vi "Chain6.vi"(7 "Name (\"\" to Use UUID)":string="CSM-Module") -> ()   [LabVIEW 2017, in "CSM-Testcase.lvlib"]
doc: "Creates a template for a CSM module without a user interface.\n\n> [!NOTE] CSM Name Rules\n> - The CSM module name must be unique to avoid entering the \"Critical Error\" state.\n> - If the input is \"\", a UUID will be used as the module name. This module will operate in independent mode and will not be listed in the module list.\n> - If the input ends with '#', the module will run in work mode. Modules with the same name will share the same message queue. External messages will be handled by the idle module.\n\n> [!NOTE] CSM Initialization State\n> - The default value is \"Macro: Initialize\", consistent with the JKISM state machine.\n> - This state is typically not modified and is provided to facilitate external programmatic changes to the initialization state.\n\n\n-- <b>Controls</b> --\n- <b>Name (\"\" to Use UUID)</b>: CSM Module Name\n- <b>Init State(\"Macro: Initialize\")</b>: Initialization State, default is \"Macro: Initialize\""
uses:
  CSM-Testcase.lvlib
  src/user.lib/_NEVSTOP/Communicable State Machine(CSM)/AdvanceAPI/CSM - Revert Arguments-Safe String.vi
  src/user.lib/_NEVSTOP/Communicable State Machine(CSM)/AdvanceAPI/CSM - Make String Arguments Safe.vi
  src/user.lib/_NEVSTOP/Communicable State Machine(CSM)/AdvanceAPI/CSM - Break Down Multiple States String.vi
  src/user.lib/_NEVSTOP/Communicable State Machine(CSM)/AdvanceAPI/CSM - Keywords.vi
  src/user.lib/_NEVSTOP/Communicable State Machine(CSM)/_Shared/Trim Single-line Text.vi
  src/user.lib/_NEVSTOP/Communicable State Machine(CSM)/_Polymophic/Build No-Reply Asynchronous Message with Arguments.vi
  src/user.lib/_NEVSTOP/Communicable State Machine(CSM)/_Polymophic/Build Asynchronous Message with Arguments.vi
  src/user.lib/_NEVSTOP/Communicable State Machine(CSM)/_Polymophic/Build Register Message.vi
  src/user.lib/_NEVSTOP/Communicable State Machine(CSM)/_Polymophic/Build Interrupt Broadcast Message.vi
  src/user.lib/_NEVSTOP/Communicable State Machine(CSM)/Communicable State Machine.lvlib
panel:
  out "Error Occurred":errorcluster
  out "State History":string
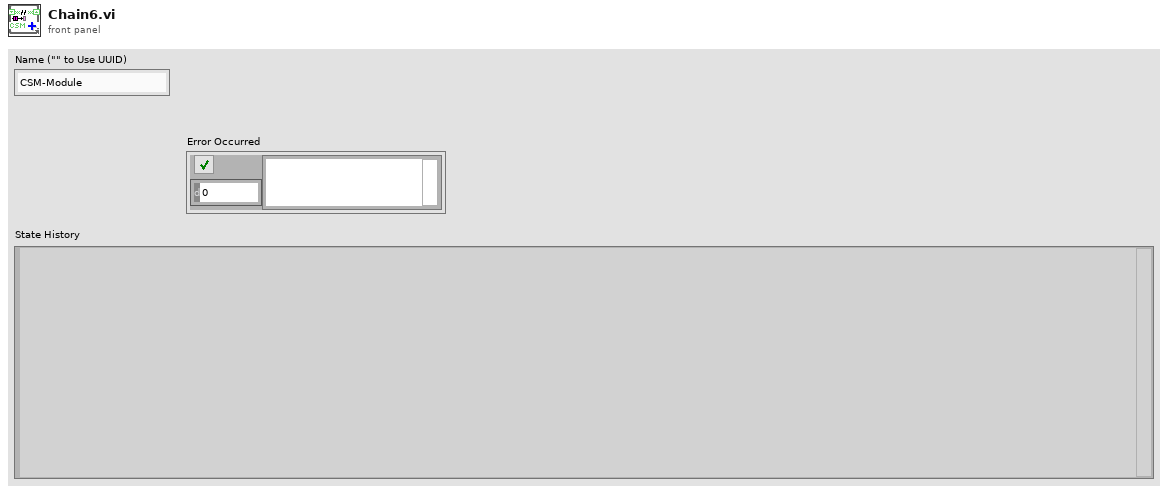
[diagram p1: front panel]
types:
  T1 = cluster{"Arguments":string, "Response":string, "error":errorcluster}
  T2 = enum32{"Invalid", "Standard", "Closed", "Hidden", "Minimized", "Maximized"}
  T3 = enum32{"invalid app kind", "Development System", "Run Time System", "Student Edition", "Embedded LabVIEW", "Evaluation", "Custom"}
  T4 = typedef "Communicable State Machine.lvlib/_CSM_Response Source Message.ctl" = cluster{"‘State":string, "’Arguments":string, "’Error":errorcluster}
  T5 = cluster{"Current VI Reference":refnum<vi>, "Close Panel on Exit?":bool}
  T6 = cluster{"Core":cluster{"Current VI Reference":refnum<vi>, "Close Panel on Exit?":bool}, "Your Boolean data":bool, "Your string data":string, "Counter":u32}
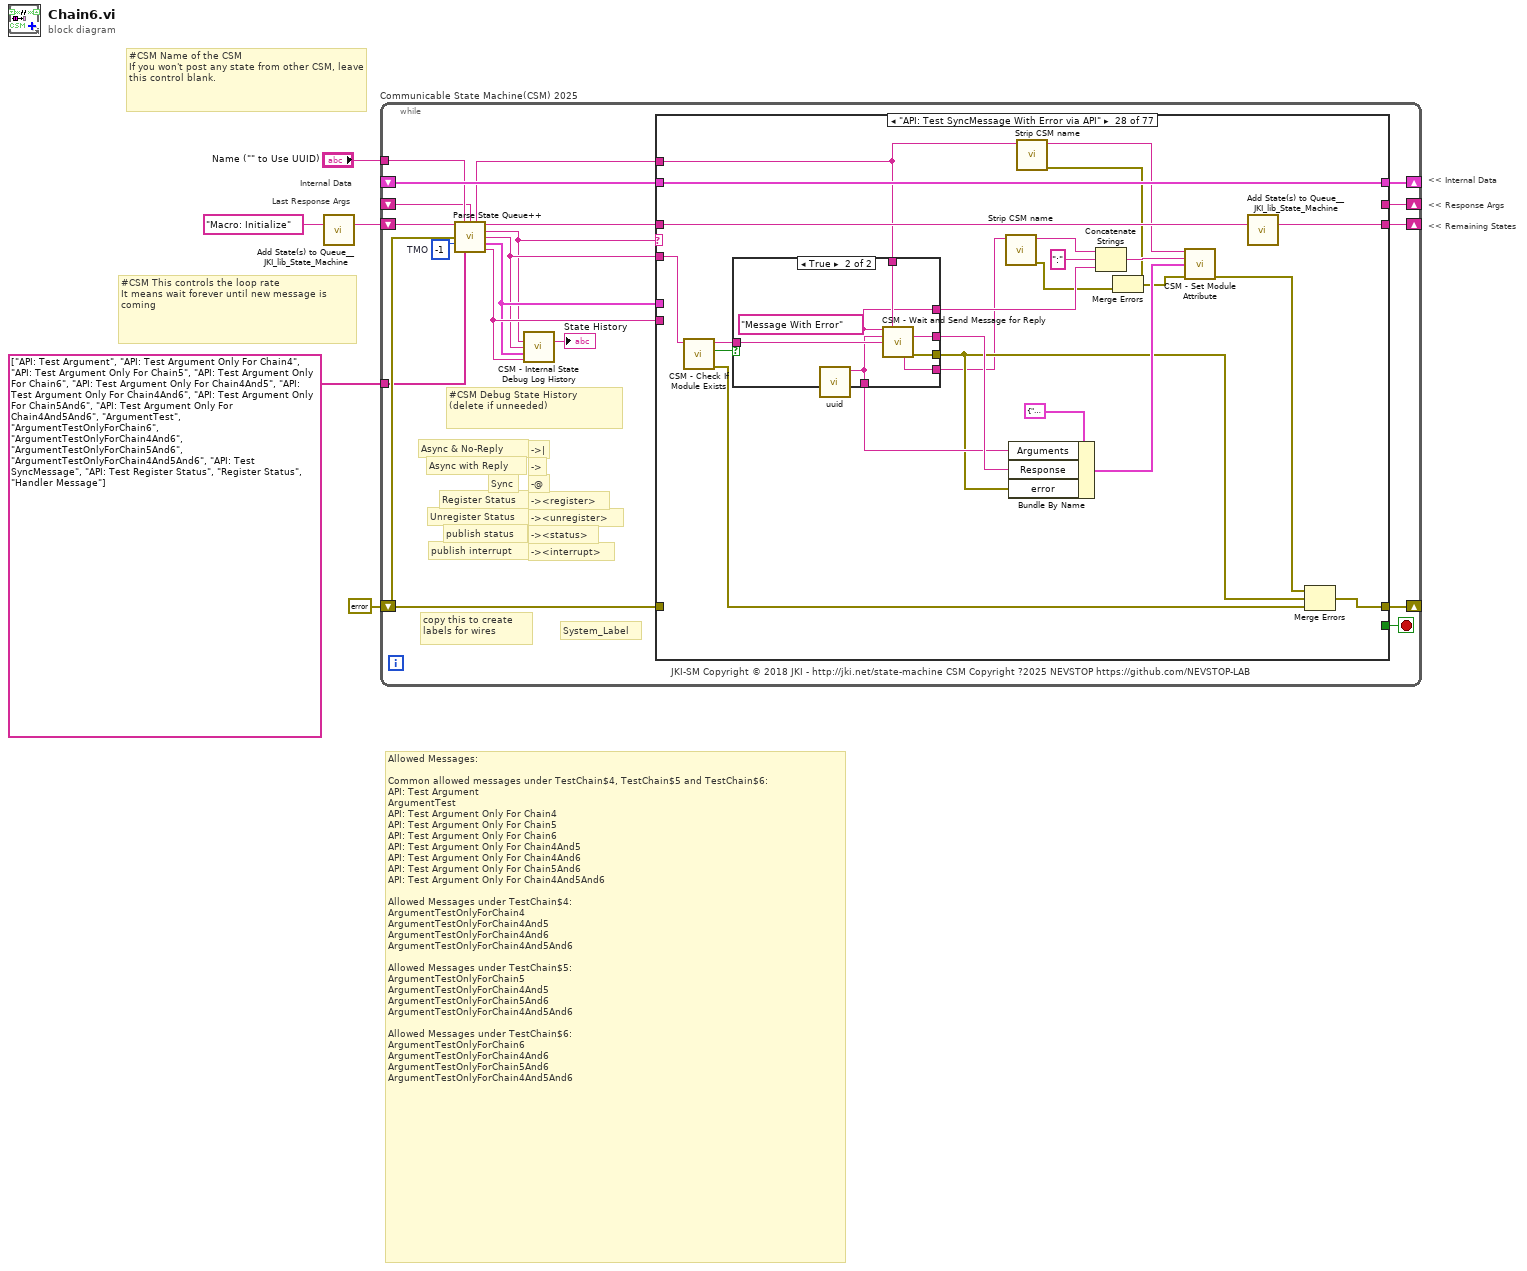
[diagram p0: block diagram]
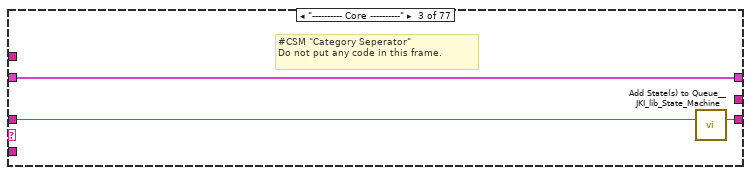
[diagram p4: hidden frame]
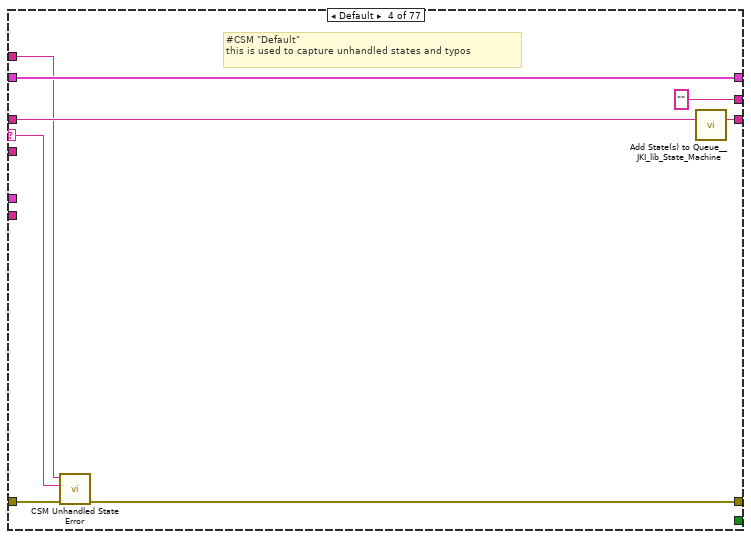
[diagram p5: hidden frame]
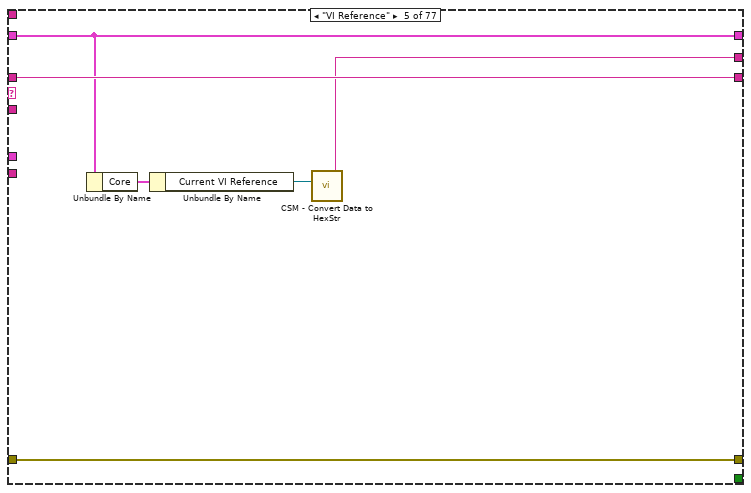
[diagram p6: hidden frame]
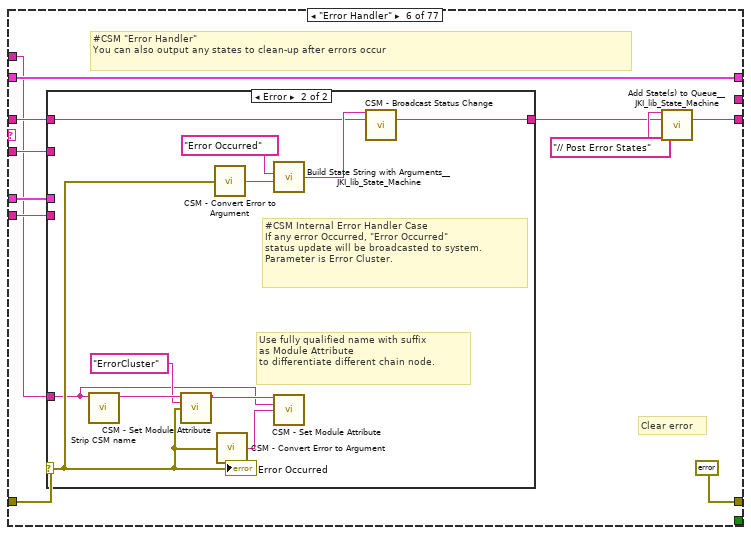
[diagram p7: hidden frame]
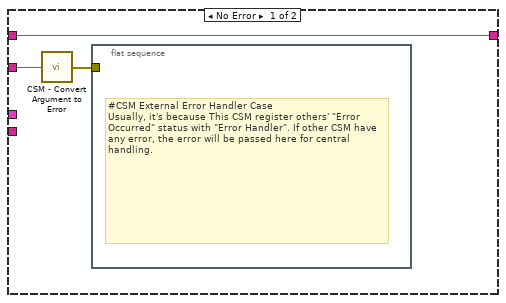
[diagram p8: hidden frame]
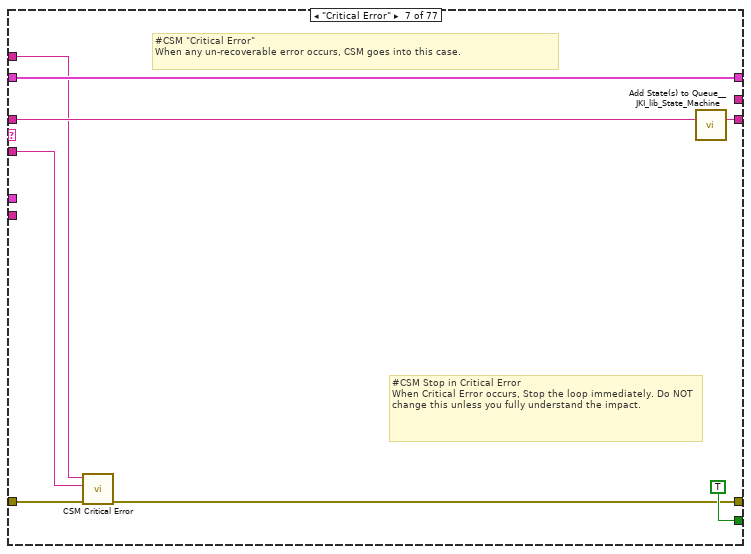
[diagram p9: hidden frame]
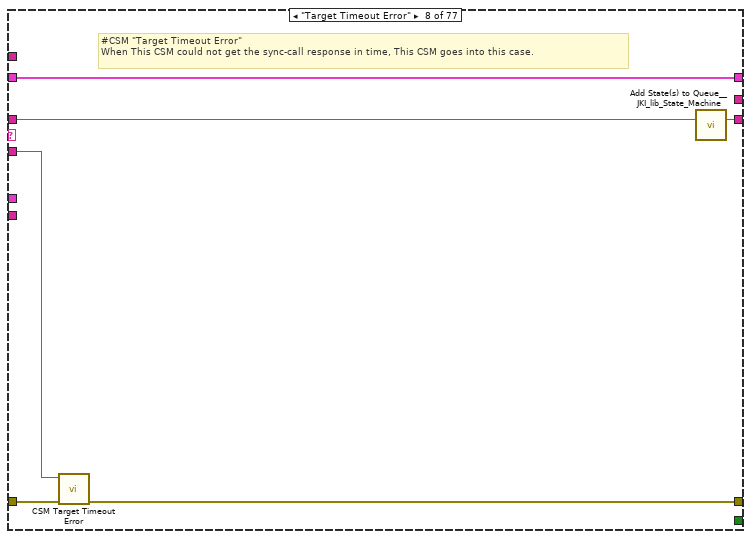
[diagram p10: hidden frame]
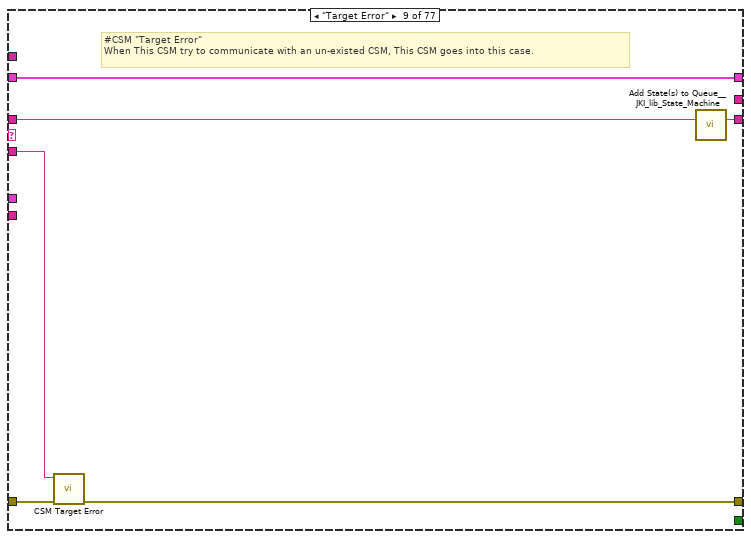
[diagram p11: hidden frame]
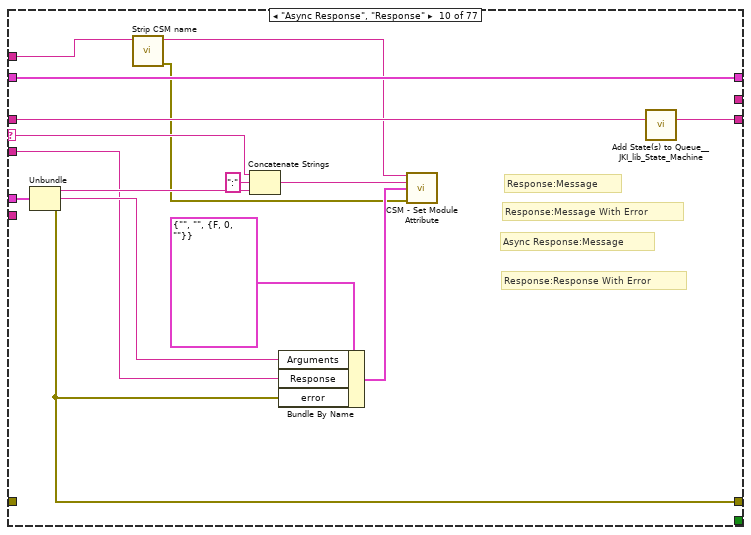
[diagram p12: hidden frame]
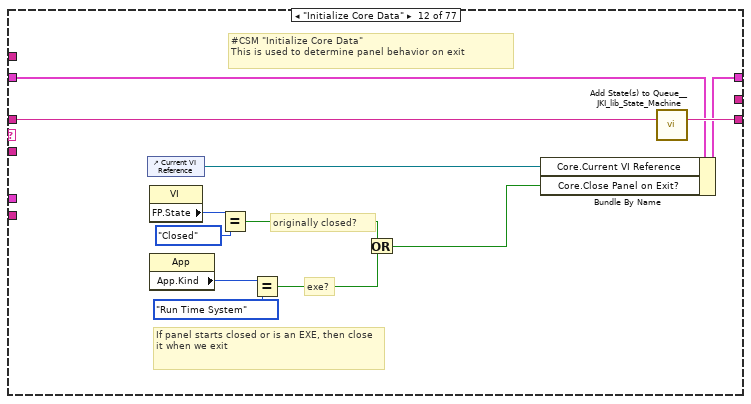
[diagram p14: hidden frame]
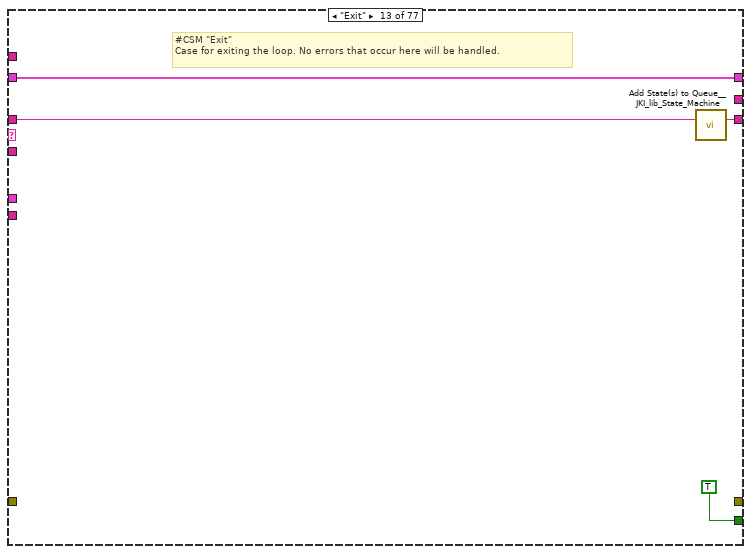
[diagram p15: hidden frame]
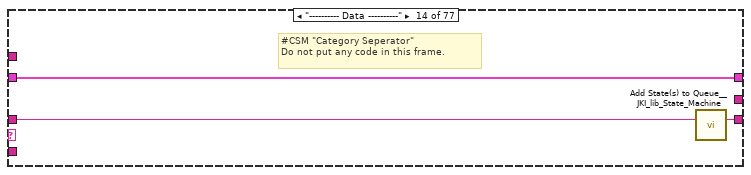
[diagram p16: hidden frame]
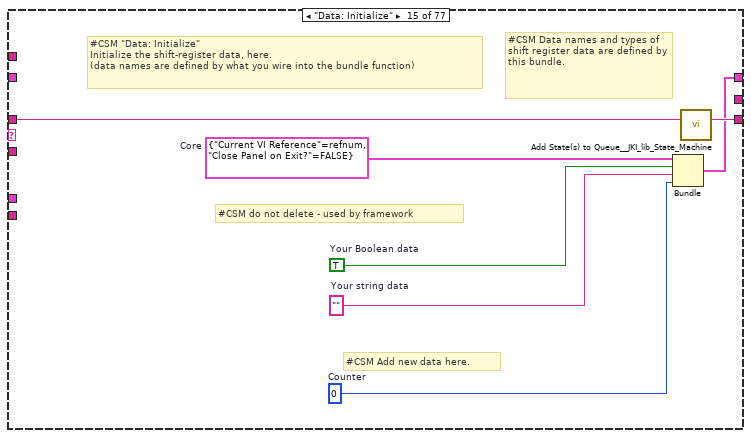
[diagram p17: hidden frame]
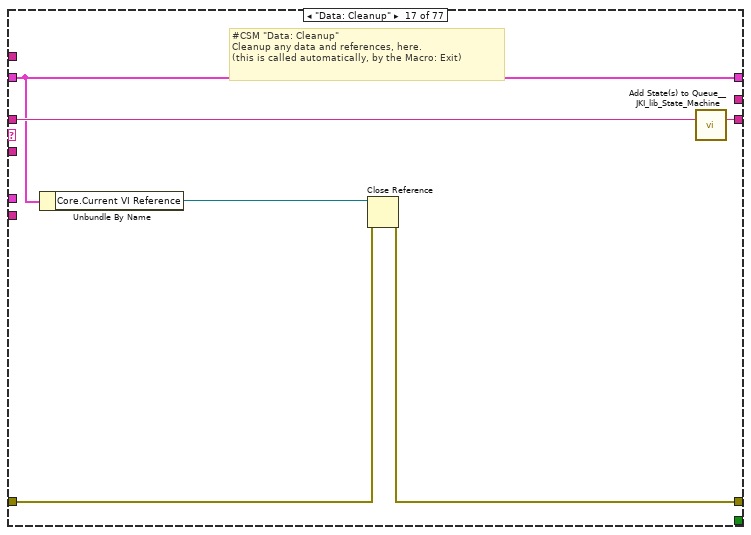
[diagram p19: hidden frame]
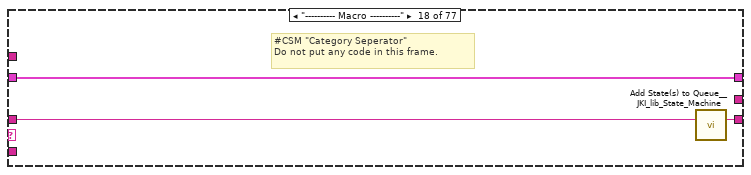
[diagram p20: hidden frame]
diagram:
  # "Allowed Messages:\n\nCommon allowed messages under TestChain$4, TestChain$5 and TestChain$6:\nAPI: Test Argument\nArgumentTest\nAPI: Test Argument Only For Chain4\nAPI: Test Argument Only For Chain5\nAPI: Test Argument Only For Chain6\nAPI: Test Argument Only For Chain4And5\nAPI: Test Argument Only For Chain4And6\nAPI: Test Argument Only For Chain5And6\nAPI: Test Argument Only For Chain4And5And6\n\nAllowed Messages under TestChain$4:\nArgumentTestOnlyForChain4\nArgumentTestOnlyForChain4And5\nArgumentTestOnlyForChain4And6\nArgumentTestOnlyForChain4And5And6\n\nAllowed Messages under TestChain$5:\nArgumentTestOnlyForChain5\nArgumentTestOnlyForChain4And5\nArgumentTestOnlyForChain5And6\nArgumentTestOnlyForChain4And5And6\n\nAllowed Messages under TestChain$6:\nArgumentTestOnlyForChain6\nArgumentTestOnlyForChain4And6\nArgumentTestOnlyForChain5And6\nArgumentTestOnlyForChain4And5And6"
  # "Last Response Args"
  # "Internal Data"
  # "#CSM Name of the CSM\nIf you won't post any state from other CSM, leave this control blank."
  # "#CSM This controls the loop rate\nIt means wait forever until new message is coming"
  # "<< Internal Data"
  # "<< Response Args"
  # "<< Remaining States"
  n1 = call <vilib>:"Add State(s) to Queue__JKI_lib_State_Machine.vi"("State(s) in (\"\")"="Macro: Initialize" ("Init State(\"Macro: Initialize\")")) -> ("States Out"=w5:string)  [unwired: 14 in]
  n2 = while "Communicable State Machine(CSM) 2025" {
    shift-right: [w19] -> _
    shift-left: _ -> [w18]
    shift-right: [w22] -> _
    shift-left: errorcluster {"status"=FALSE, "code"=0, "source"=""} ("error out") -> [w8]
    shift-right: [w21] -> _
    shift-left: w5 -> [w23]
    tunnel: "Name (\"\" to Use UUID)" -> [w15]
    shift-right: [w16] -> _
    shift-left: _ -> [w10]
    tunnel: string[] ["API: Test Argument", "API: Test Argument Only For Chain4", "API: Test Argument Only For Chain5", "API: Test Argument Only For Chain6", "API: Test Argument Only For Chain4And5", "API: Test Argument Only For Chain4And6", "API: Test Argument Only For Chain5And6", "API: Test Argument Only For Chain4And5And6", "ArgumentTest", "ArgumentTestOnlyForChain6", "ArgumentTestOnlyForChain4And6", "ArgumentTestOnlyForChain5And6", "ArgumentTestOnlyForChain4And5And6", "API: Test SyncMessage", "API: Test Register Status", "Register Status", "Handler Message"] ("Allowed Messages (Empty for All)") -> [w6]
    stop <- w20 stop-if-true
    w17 = -1  # TMO
    # "#CSM Debug State History\n(delete if unneeded)"
    # "-><interrupt>"
    # "-><status>"
    # "-><unregister>"
    # "-><register>"
    # "-@"
    # "->"
    # "->|"
    # "publish interrupt"
    # "publish status"
    # "Unregister Status"
    # "Register Status"
    # "Sync"
    # "Async with Reply"
    # "Async & No-Reply"
    # "JKI-SM Copyright © 2018 JKI - http://jki.net/state-machine CSM Copyright ?2025 NEVSTOP https://github.com/NEVSTOP-LAB"
    # "copy this to create labels for wires"
    # "System_Label"
    n3 = call "Parse State Queue++.vi"("State Queue"=w23, "Name (\"\" to Use UUID)"=w15, "Response Arguments"=w10, "Previous Error"=w8, "Dequeue (1 ms)"=w17, "Allowed Messages (Empty for All)"=w6) -> ("Name Used"=w9:string, "Remaining States"=w24:string, "Current State"=w11:string, "Arguments"=w12:string, "Additional Information"=w13:T4, "Source CSM"=w14:string)  [unwired: 4 in]
    n4 = call "CSM - Internal State Debug Log History.vi"("State"=w11, "Arguments (\"\")"=w12, ">> Response Source Message >>"=w13, "Source (\"\")"=w14) -> ("Debug Log"=→"State History":string)  [unwired: 11 in]
    n5 = case shown="\"API: Test SyncMessage With Error via API\"" w11 {
      selector: w11 -> [_ _ _ w35 _ _ _ _ _ w102 _ _ _ _ _ _ _ _ _ _ _ _ _ _ _ _ _ _ _ _ _ _ _ w387 _ _ _ _ _ _ _ _ _ _ _ _ _ _ _ _ _ _ _ _ _ _ w579 _ _ _ _ _ _ _ _ _ _ w647 _ _ _ w672 _ w694 w701 w717 _]
      tunnel: w24 -> [w25 w28 w31 w39 w44 w50 w78 w84 w90 w106 w108 w120 w124 w127 w134 w136 w142 w145 w149 w155 w169 w189 w218 w222 w226 w238 w266 w297 w312 w324 w336 w350 w373 w405 w421 w434 w441 w448 w455 w462 w469 w476 w483 w490 w497 w504 w511 w523 w532 w542 w552 w562 w566 w571 w574 w578 w585 w592 w595 w608 w614 w620 w624 w629 w633 w637 w641 w651 w655 w663 w669 w677 w687 w696 w706 w722 w734]
      tunnel: w12 -> [_ _ _ _ _ w49 w74 w81 w87 w96 _ _ _ _ _ _ _ _ _ _ w156 w176 w201 _ w229 w241 w269 w300 w315 w327 w339 w353 w369 w403 w424 w431 w438 w445 w452 w459 w466 w473 w480 w487 w494 w501 w508 w515 _ w534 w543 w553 w564 _ _ w575 _ w588 w597 _ w610 w616 w622 w627 w632 w636 w640 w646 w654 w661 w667 w674 w683 w695 w700 w712 _]
      tunnel: w18 -> [w26 w27 w29 w37 w43 w55 w76 w82 w88 w104 w107 w114 w122 w125 _ w135 w137 w143 w147 w153 w171 w191 w220 w221 w230 w242 w270 w301 w316 w328 w340 w354 w376 w408 w425 w436 w443 w450 w457 w464 w471 w478 w485 w492 w499 w506 w513 w521 w530 w540 w550 w560 w565 w569 w572 w576 w586 w593 w599 w609 w615 w621 w626 w631 w634 w638 w642 w652 w656 w662 w668 w678 w681 w697 w707 w714 w732]
      tunnel: [_ _ _ w32 w45 errorcluster {"status"=FALSE, "code"=0, "source"=""} ("error out") w71 w79 w85 w95 _ _ _ _ _ _ w138 _ _ _ _ _ _ _ w223 w235 w263 w294 w309 w321 w333 w346 w370 w389 w418 w435 w442 w449 w456 w463 w470 w477 w484 w491 w498 w505 w512 w517 w526 w536 w547 w557 _ _ _ _ w581 _ _ w601 _ _ w625 w630 w635 w639 w643 w645 w657 w658 w664 w671 w684 w690 w702 w718 _] -> w22
      tunnel: w8 -> [_ _ _ w33 w45 w53 w72 w80 w86 _ _ _ _ _ _ _ w139 _ _ _ _ _ _ _ _ _ _ _ _ _ _ _ _ _ _ w435 w442 w449 w456 w463 w470 w477 w484 w491 w498 w505 w512 _ _ _ _ _ _ _ _ _ _ _ _ _ _ _ w625 w630 w635 w639 w643 w653 w657 w659 w665 w679 w688 w698 w708 w723 _]
      tunnel: [w25 w28 w30 w38 w44 w51 w77 w83 w89 w105 w108 w119 w123 w126 w133 w136 w141 w144 w148 w154 w170 w190 w219 w222 w227 w239 w267 w298 w313 w325 w337 w351 w374 w406 w422 w433 w440 w447 w454 w461 w468 w475 w482 w489 w496 w503 w510 w522 w531 w541 w551 w561 w566 w570 w573 w577 w587 w589 w594 w606 w611 w617 w623 w628 w633 w637 w641 w651 w655 w663 w669 w677 w687 w696 w706 w722 w733] -> w21
      tunnel: [_ _ _ _ _ _ TRUE _ _ _ _ _ TRUE _ _ _ _ _ _ _ _ _ _ _ _ _ _ _ _ _ _ _ _ _ _ _ _ _ _ _ _ _ _ _ _ _ _ _ _ _ _ _ _ _ _ _ _ _ _ _ _ _ _ _ _ _ _ _ _ _ _ _ _ _ _ _ _] -> w20
      tunnel: [w26 w27 w29 w37 w43 w55 w76 w82 w88 w104 w107 w118 w122 w125 w132 w135 w137 w143 w147 w153 w171 w191 w220 w221 w230 w242 w270 w301 w316 w328 w340 w354 w376 w408 w425 w436 w443 w450 w457 w464 w471 w478 w485 w492 w499 w506 w513 w521 w530 w540 w550 w560 w565 w569 w572 w576 w586 w593 w599 w609 w615 w621 w626 w631 w634 w638 w642 w652 w656 w662 w668 w678 w681 w697 w707 w713 w730] -> w19
      tunnel: w14 -> [_ _ _ _ _ w48 _ _ _ _ _ _ _ _ _ _ _ _ _ _ _ _ _ _ _ _ _ _ _ _ _ _ _ _ _ _ _ _ _ _ _ _ _ _ _ _ _ _ _ _ _ _ _ _ _ _ _ _ _ _ _ _ _ _ _ _ _ _ _ _ _ _ _ _ _ _ _]
      tunnel: w13 -> [_ _ _ _ _ w47 _ _ _ w103 _ _ _ _ _ _ _ _ _ _ _ _ _ _ _ _ _ _ _ _ _ _ _ _ _ _ _ _ _ _ _ _ _ _ _ _ _ _ _ _ _ _ _ _ _ _ _ _ _ _ _ _ _ _ _ _ _ _ _ _ _ _ _ _ _ _ _]
      tunnel: [_ _ _ "" w40 _ _ _ _ _ _ _ _ _ _ _ _ _ _ _ _ _ _ _ _ _ _ _ _ _ _ _ _ w390 _ _ _ _ _ _ _ _ _ _ _ _ _ _ _ _ _ _ w563 _ _ w575 w580 _ _ _ _ _ w622 w627 w632 w636 w640 w646 w654 w661 w667 _ w683 w695 w700 _ _] -> w16
      tunnel: w9 -> [_ _ _ w34 _ w46 w73 _ _ w93 _ _ _ _ _ _ _ _ _ _ _ _ _ _ _ _ w254 w285 _ _ _ w347 _ w393 _ _ _ _ _ _ _ _ _ _ _ _ _ w519 w528 w538 w549 w559 _ _ _ _ w582 _ _ w603 _ _ _ _ _ _ _ w650 _ _ _ w676 w680 w693 w705 w721 _]
      frame "", "Idle" {
        # "#CSM \"Idle/Event Handler\"\nexecutes when the state queue is empty"
      }
      frame "CSM Documentation" {
        # "#CSM State Syntax\n\n// Comment line, all text to the right of “//” will be ignored\n// Local Message Example\nDoSth: DoA >> Arguments\n\n// Sync Call Example\nAPI: xxxx >> Arguments -@ TargetModule\n\n// Async Call Example\nAPI: xxxx >> Arguments -> TargetModule\n\n// Async Call without Reply Example\nAPI: xxxx >> Arguments ->| TargetModule\n\n// Broadcast normal status:\nStatus >> StatusArguments  -><status>\n\n// Broadcast Interrupt status:\nInterrupt >> StatusArguments  -><interrupt>\n\n// Register Source Module's status to Handler Module\nStatus@Source Module >> Handler Module@Handler Module -><register>\n\n// Unegister Source Module's status\nStatus@Source Module >> Handler Module -><unregister>"
        # "#CSM README FIRST\n\nCommunicable State Machine(CSM) is a LabVIEW application framework that builds upon JKI State Machine(JKISM). It follows the pattern of JKISM and extends the keywords to describe message communication between modules, including concepts such as Sync-Message, Async-Message, Subscription/Unsubscription of status - essential elements for creating reusable code modules. For more information, please visit the CSM wiki: https://nevstop-lab.github.io/CSM-Wiki/\n\nFor instructions on JKI State Machine, visit: \n    http://jki.net/state-machine/\nFor information about CSM, visit: \n    https://github.com/NEVSTOP-LAB"
        # "#CSM \"Documentation\"\nCase for holding CSM Documenation"
      }
      frame "---------- Core ----------" {
        # "#CSM \"Category Seperator\"\nDo not put any code in this frame."
        n6 = call <vilib>:"Add State(s) to Queue__JKI_lib_State_Machine.vi"("State(s) in (\"\")"=w31) -> ("States Out"=w30:string)  [unwired: 14 in]
      }
      frame Default {
        # "#CSM \"Default\"\nthis is used to capture unhandled states and typos"
        n7 = call "CSM Unhandled State Error.vi"("error in (no error)"=w33, "Undefined State"=w35, "CSM Name"=w34) -> ("error out"=w32:errorcluster)  [unwired: 8 in]
        n8 = call <vilib>:"Add State(s) to Queue__JKI_lib_State_Machine.vi"("State(s) in (\"\")"=w39) -> ("States Out"=w38:string)  [unwired: 14 in]
      }
      frame "VI Reference" {
        n9 = Unbundle By Name(w43) -> ("Core"=w42:T5)
        n10 = Unbundle By Name(w42) -> ("Current VI Reference"=w41:refnum<vi>)
        n11 = call "CSM - Convert Data to HexStr.vi"("Variant"=w41) -> ("HEX String (0-9,A-F)"=w40:string)  [unwired: 8 in]
      }
      frame "Error Handler" {
        # "#CSM \"Error Handler\"\nYou can also output any states to clean-up after errors occur"
        # "Clear error"
        n12 = case shown="Error" w53 {
          selector: w53 -> [_ w61]
          tunnel: [w59 w67] -> w52
          tunnel: w50 -> [w59 w66]
          tunnel: w49 -> [w58 _]
          tunnel: w48 -> [_ _]
          tunnel: w47 -> [_ _]
          tunnel: w46 -> [_ w60]
          frame No Error {
            n13 = call "CSM - Convert Argument to Error.vi"("Argument"=w58) -> ("Error"=w57:errorcluster)  [unwired: 4 in]
            n14 = flat-sequence {
              tunnel: w57 -> [_]
              frame #0 {
                # "#CSM External Error Handler Case\nUsually, it's because This CSM register others' \"Error Occurred\" status with \"Error Handler\". If other CSM have any error, the error will be passed here for central handling."
              }
            }
          }
          frame Error {
            # "Use fully qualified name with suffix \nas Module Attribute  \nto differentiate different chain node."
            # "#CSM Internal Error Handler Case \nIf any error Occurred, \"Error Occurred\" \nstatus update will be broadcasted to system.\nParameter is Error Cluster."
            n15 = call "Strip CSM name.vi"("CSM name"=w60) -> ("CSM name core"=w65:string)  [unwired: 7 in, 3 out]
            n16 = call "CSM - Set Module Attribute.vi"("CSM Name"=w65, "Attribute"="ErrorCluster", "Value"=w61) -> ("CSM Name (Dup)"=w62:string)  [unwired: 9 in, 3 out]
            n17 = call "CSM - Convert Error to Argument.vi"("Error"=w61) -> ("Argument"=w69:string)  [unwired: 4 in]
            n18 = call "CSM - Convert Error to Argument.vi"("Error"=w61) -> ("Argument"=w63:string)  [unwired: 4 in]
            n19 = call <vilib>:"Build State String with Arguments__JKI_lib_State_Machine.vi"("Arguments (\"\")"=w69, "State"="Error Occurred" ("Status with Arguments")) -> ("State with Arguments"=w68:string)  [unwired: 4 in]
            n20 = call "CSM - Set Module Attribute.vi"("CSM Name"=w62, "Attribute"=w60, "Value"=w63) -> ()  [unwired: 9 in, 4 out]
            n21 = call "CSM - Broadcast Status Change.vi"("Status With Arguments"=w68, "State Queue"=w66) -> ("Remaining States"=w67:string)  [unwired: 13 in]
            "Error Occurred" <- w61
          }
        }
        n22 = call <vilib>:"Add State(s) to Queue__JKI_lib_State_Machine.vi"("State(s) in Front (\"\")"="// Post Error States", "State(s) in (\"\")"=w52) -> ("States Out"=w51:string)  [unwired: 13 in]
      }
      frame "Critical Error" {
        # "#CSM \"Critical Error\"\nWhen any un-recoverable error occurs, CSM goes into this case."
        # "#CSM Stop in Critical Error\nWhen Critical Error occurs, Stop the loop immediately. Do NOT change this unless you fully understand the impact."
        n23 = call "CSM Critical Error.vi"("error in (no error)"=w72, "Arugments (As Reason)"=w74, "CSM Name"=w73) -> ("error out"=w71:errorcluster)  [unwired: 8 in]
        n24 = call <vilib>:"Add State(s) to Queue__JKI_lib_State_Machine.vi"("State(s) in (\"\")"=w78) -> ("States Out"=w77:string)  [unwired: 14 in]
      }
      frame "Target Timeout Error" {
        # "#CSM \"Target Timeout Error\"\nWhen This CSM could not get the sync-call response in time, This CSM goes into this case."
        n25 = call "CSM Target Timeout Error.vi"("error in (no error)"=w80, "Arguments (As CSM Name)"=w81) -> ("error out"=w79:errorcluster)  [unwired: 9 in]
        n26 = call <vilib>:"Add State(s) to Queue__JKI_lib_State_Machine.vi"("State(s) in (\"\")"=w84) -> ("States Out"=w83:string)  [unwired: 14 in]
      }
      frame "Target Error" {
        # "#CSM \"Target Error\"\nWhen This CSM try to communicate with an un-existed CSM, This CSM goes into this case."
        n27 = call "CSM Target Error.vi"("error in (no error)"=w86, "Arguments (As CSM Name)"=w87) -> ("error out"=w85:errorcluster)  [unwired: 9 in]
        n28 = call <vilib>:"Add State(s) to Queue__JKI_lib_State_Machine.vi"("State(s) in (\"\")"=w90) -> ("States Out"=w89:string)  [unwired: 14 in]
      }
      frame "Async Response", "Response" {
        # "Response:Response With Error"
        # "Response:Message With Error"
        # "Async Response:Message"
        # "Response:Message"
        n29 = Unbundle(w103) -> ("‘State"=w101:string, "’Arguments"=w97:string, "’Error"=w95:errorcluster)
        n30 = call "Strip CSM name.vi"("CSM name"=w93) -> ("error out"=w91:errorcluster, "CSM name core"=w92:string)  [unwired: 7 in, 2 out]
        n31 = Concatenate Strings(w102, ":" ("string"), w101) -> (w99:string)
        n32 = Bundle By Name(cluster=T1 {"Arguments"="", "Response"="", "error"={"status"=FALSE, "code"=0, "source"=""}}, "Arguments"=w97, "Response"=w96, "error"=w95) -> (w94:T1)
        n33 = call "CSM - Set Module Attribute.vi"("CSM Name"=w92, "Attribute"=w99, "Value"=w94, "Error In"=w91) -> ()  [unwired: 8 in, 4 out]
        n34 = call <vilib>:"Add State(s) to Queue__JKI_lib_State_Machine.vi"("State(s) in (\"\")"=w106) -> ("States Out"=w105:string)  [unwired: 14 in]
      }
      frame "Async Message Posted" {
        # "#CSM \"Async Message Posted\"\nAfter Async Message is posted (-> or ->| ), CSM goes to this state for post-action.\nYou can use Argument - State to tell which Async Message is called."
      }
      frame "Initialize Core Data" {
        # "#CSM \"Initialize Core Data\"\nThis is used to determine panel behavior on exit"
        # "originally closed?"
        # "exe?"
        # "If panel starts closed or is an EXE, then close it when we exit"
        n35 = control-ref of="Current VI Reference"() -> (w112:refnum<vi>)
        n36 = property class="VI"() -> ("FP.State"=w111:T2)  [unwired: 2 in, 2 out]
        n37 = property class="App"() -> ("App.Kind"=w117:T3)  [unwired: 2 in, 2 out]
        n38 = Equal?(x=w111, y=T2."Closed" ("Front Panel Window:State")) -> (x = y?=w109:bool)
        n39 = Equal?(x=w117, y=T3."Run Time System" ("Application:Kind")) -> (x = y?=w115:bool)
        n40 = Or(x=w109, y=w115) -> (x .or. y?=w113:bool)
        n41 = Bundle By Name(cluster=w114, "Core.Current VI Reference"=w112, "Core.Close Panel on Exit?"=w113) -> (w118:T6)
        n42 = call <vilib>:"Add State(s) to Queue__JKI_lib_State_Machine.vi"("State(s) in (\"\")"=w120) -> ("States Out"=w119:string)  [unwired: 14 in]
      }
      frame "Exit" {
        # "#CSM \"Exit\"\nCase for exiting the loop. No errors that occur here will be handled."
        n43 = call <vilib>:"Add State(s) to Queue__JKI_lib_State_Machine.vi"("State(s) in (\"\")"=w124) -> ("States Out"=w123:string)  [unwired: 14 in]
      }
      frame "---------- Data ----------" {
        # "#CSM \"Category Seperator\"\nDo not put any code in this frame."
        n44 = call <vilib>:"Add State(s) to Queue__JKI_lib_State_Machine.vi"("State(s) in (\"\")"=w127) -> ("States Out"=w126:string)  [unwired: 14 in]
      }
      frame "Data: Initialize" {
        w128 = u32 0  # Counter
        w129 = T5 {"Current VI Reference"=refnum, "Close Panel on Exit?"=FALSE}  # Core
        w131 = TRUE  # Your Boolean data
        w130 = ""  # Your string data
        # "#CSM \"Data: Initialize\"\nInitialize the shift-register data, here.\n(data names are defined by what you wire into the bundle function)"
        # "#CSM do not delete - used by framework"
        # "#CSM Add new data here."
        # "#CSM Data names and types of shift register data are defined by this bundle."
        n45 = Bundle("Core"=w129, "Your Boolean data"=w131, "Your string data"=w130, "Counter"=w128) -> (w132:T6)  [unwired: 1 in]
        n46 = call <vilib>:"Add State(s) to Queue__JKI_lib_State_Machine.vi"("State(s) in (\"\")"=w134) -> ("States Out"=w133:string)  [unwired: 14 in]
      }
      frame "Data: Update Indicators" {
      }
      frame "Data: Cleanup" {
        # "#CSM \"Data: Cleanup\"\nCleanup any data and references, here.\n(this is called automatically, by the Macro: Exit)"
        n47 = Unbundle By Name(w137) -> ("Core.Current VI Reference"=w140:refnum<vi>)
        n48 = Close Reference(reference=w140, error in (no error)=w139) -> (error out=w138:errorcluster)
        n49 = call <vilib>:"Add State(s) to Queue__JKI_lib_State_Machine.vi"("State(s) in (\"\")"=w142) -> ("States Out"=w141:string)  [unwired: 14 in]
      }
      frame "---------- Macro ----------" {
        # "#CSM \"Category Seperator\"\nDo not put any code in this frame."
        n50 = call <vilib>:"Add State(s) to Queue__JKI_lib_State_Machine.vi"("State(s) in (\"\")"=w145) -> ("States Out"=w144:string)  [unwired: 14 in]
      }
      frame "Macro: Initialize" {
        # "#CSM \"Macro: Initialize\"\nInitialization Macro (This is called once, when the VI starts)"
        n51 = call <vilib>:"Add State(s) to Queue__JKI_lib_State_Machine.vi"("State(s) in Front (\"\")"="Data: Initialize\nInitialize Core Data\nData: Update Indicators", "State(s) in (\"\")"=w149) -> ("States Out"=w148:string)  [unwired: 13 in]
      }
      frame "Macro: Exit" {
        # "#CSM \"Macro: Exit\"\nExit Macro (This is called once, when the VI exits)"
        n52 = call <vilib>:"Add State(s) to Queue__JKI_lib_State_Machine.vi"("State(s) in Front (\"\")"="//Exit Sub-Modules ", "State(s) at Back (\"\")"="Data: Cleanup\nExit") -> ("States Out"=w151:string)  [unwired: 13 in]
        n53 = call <vilib>:"Add State(s) to Queue__JKI_lib_State_Machine.vi"("State(s) in Front (\"\")"=w151, "State(s) in (\"\")"=w155) -> ("States Out"=w154:string)  [unwired: 13 in]
      }
      frame "Macro: Test MacroWithSubMessages" {
        w157 = "SubMessage2" ("State With Arguments")
        w159 = "SubMessage1" ("State With Arguments")
        n54 = call "uuid.vi"() -> ("UUID"=w158:string)  [unwired: 11 in]
        n55 = call "uuid.vi"() -> ("UUID"=w160:string)  [unwired: 11 in]
        n56 = Concatenate Strings(w159, w160) -> (w161:string)
        n57 = Concatenate Strings(w157, w158) -> (w162:string)
        n58 = call <vilib>:"Build State String with Arguments__JKI_lib_State_Machine.vi"("Arguments (\"\")"=w156, "State"="SubMessage3" ("State With Arguments")) -> ("State with Arguments"=w164:string)  [unwired: 4 in]
        n59 = call <vilib>:"Build State String with Arguments__JKI_lib_State_Machine.vi"("Arguments (\"\")"=w161, "State"=w159) -> ("State with Arguments"=w166:string)  [unwired: 4 in]
        n60 = call <vilib>:"Build State String with Arguments__JKI_lib_State_Machine.vi"("Arguments (\"\")"=w162, "State"=w157) -> ("State with Arguments"=w165:string)  [unwired: 4 in]
        n61 = Build Array(w166, w165, w164) -> (w163:string[])
        n62 = call "CSM - Compact Multiple States.vi"("Multiple States"=w163) -> ("States"=w168:string)  [unwired: 9 in]
        n63 = call <vilib>:"Add State(s) to Queue__JKI_lib_State_Machine.vi"("State(s) in Front (\"\")"=w168, "State(s) in (\"\")"=w169) -> ("States Out"=w170:string)  [unwired: 13 in]
      }
      frame "Macro: Test MacroWithSubAndPostMessages" {
        w175 = "PostMessage1" ("State With Arguments")
        w177 = "SubMessage2" ("State With Arguments")
        w179 = "SubMessage1" ("State With Arguments")
        n64 = call "uuid.vi"() -> ("UUID"=w178:string)  [unwired: 11 in]
        n65 = call "uuid.vi"() -> ("UUID"=w174:string)  [unwired: 11 in]
        n66 = call "uuid.vi"() -> ("UUID"=w180:string)  [unwired: 11 in]
        n67 = Concatenate Strings(w175, w174) -> (w173:string)
        n68 = Concatenate Strings(w179, w180) -> (w181:string)
        n69 = Concatenate Strings(w177, w178) -> (w182:string)
        n70 = call <vilib>:"Build State String with Arguments__JKI_lib_State_Machine.vi"("Arguments (\"\")"=w176, "State"="SubMessage3" ("State With Arguments")) -> ("State with Arguments"=w184:string)  [unwired: 4 in]
        n71 = call <vilib>:"Build State String with Arguments__JKI_lib_State_Machine.vi"("Arguments (\"\")"=w173, "State"=w175) -> ("State with Arguments"=w172:string)  [unwired: 4 in]
        n72 = call <vilib>:"Build State String with Arguments__JKI_lib_State_Machine.vi"("Arguments (\"\")"=w181, "State"=w179) -> ("State with Arguments"=w186:string)  [unwired: 4 in]
        n73 = call <vilib>:"Build State String with Arguments__JKI_lib_State_Machine.vi"("Arguments (\"\")"=w182, "State"=w177) -> ("State with Arguments"=w185:string)  [unwired: 4 in]
        n74 = Build Array(w186, w185, w184) -> (w183:string[])
        n75 = call "CSM - Compact Multiple States.vi"("Multiple States"=w183) -> ("States"=w188:string)  [unwired: 9 in]
        n76 = call <vilib>:"Add State(s) to Queue__JKI_lib_State_Machine.vi"("State(s) in Front (\"\")"=w188, "State(s) in (\"\")"=w189, "State(s) at Back (\"\")"=w172) -> ("States Out"=w190:string)  [unwired: 12 in]
      }
      frame "Macro: TestMacroWithNonLocalSubMessages" {
        w205 = "PostMessage1" ("State With Arguments")
        w206 = "SubMessage2" ("State With Arguments")
        w208 = "SubMessage1" ("State With Arguments")
        n77 = Match Pattern(string=w201, regular expression="+") -> (before substring=w193:string, after substring=w192:string)  [unwired: 1 in, 2 out]
        n78 = call "uuid.vi"() -> ("UUID"=w204:string)  [unwired: 11 in]
        n79 = call "uuid.vi"() -> ("UUID"=w207:string)  [unwired: 11 in]
        n80 = call "uuid.vi"() -> ("UUID"=w209:string)  [unwired: 11 in]
        n81 = Concatenate Strings(w205, w204) -> (w203:string)
        n82 = Concatenate Strings(w208, w209) -> (w210:string)
        n83 = Concatenate Strings(w206, w207) -> (w211:string)
        n84 = call <vilib>:"Build State String with Arguments__JKI_lib_State_Machine.vi"("Arguments (\"\")"=w203, "State"=w205) -> ("State with Arguments"=w202:string)  [unwired: 4 in]
        n85 = call-poly "Build Message with Arguments++.vi"("State With Arguments"="SubMessage1", "Target Module (\"\")"=w192) -> ("CSM Message String"=w197:string)  [unwired: 13 in]
        n86 = call-poly "Build Message with Arguments++.vi"("State With Arguments"="SubMessage2", "Target Module (\"\")"=w192) -> ("CSM Message String"=w196:string)  [unwired: 13 in]
        n87 = call <vilib>:"Build State String with Arguments__JKI_lib_State_Machine.vi"("Arguments (\"\")"=w193, "State"="SubMessage3" ("State With Arguments")) -> ("State with Arguments"=w213:string)  [unwired: 4 in]
        n88 = call-poly "Build Message with Arguments++.vi"("State With Arguments"="Message", "Target Module (\"\")"=w192) -> ("CSM Message String"=w198:string)  [unwired: 13 in]
        n89 = call <vilib>:"Build State String with Arguments__JKI_lib_State_Machine.vi"("Arguments (\"\")"=w210, "State"=w208) -> ("State with Arguments"=w215:string)  [unwired: 4 in]
        n90 = call <vilib>:"Build State String with Arguments__JKI_lib_State_Machine.vi"("Arguments (\"\")"=w211, "State"=w206) -> ("State with Arguments"=w214:string)  [unwired: 4 in]
        n91 = Build Array(w215, w214, w213, w198, w197, w196) -> (w212:string[])
        n92 = call "CSM - Compact Multiple States.vi"("Multiple States"=w212) -> ("States"=w217:string)  [unwired: 9 in]
        n93 = call <vilib>:"Add State(s) to Queue__JKI_lib_State_Machine.vi"("State(s) in Front (\"\")"=w217, "State(s) in (\"\")"=w218, "State(s) at Back (\"\")"=w202) -> ("States Out"=w219:string)  [unwired: 12 in]
      }
      frame "---------- API ----------" {
        # "#CSM \"Category Seperator\"\nDo not put any code in this frame."
      }
      frame "API: Test SyncMessage" {
        n94 = call "CSM - Check If Module Exists.vi"("CSM Name"=w229) -> ("error out"=w223:errorcluster, "Exist?"=w224:bool, "CSM Name (Dup)"=w228:string)  [unwired: 8 in]
        n95 = case shown="True" w224 {
          tunnel: w228 -> [_ w232]
          tunnel: [_ w231] -> w225
          frame False {
          }
          frame True {
            n96 = call "uuid.vi"() -> ("UUID"=w233:string)  [unwired: 11 in]
            n97 = call-poly "Build Message with Arguments++.vi"("State With Arguments"="Message", "Arguments (\"\")"=w233, "Target Module (\"\")"=w232) -> ("CSM Message String"=w231:string)  [unwired: 12 in]
          }
        }
        n98 = call <vilib>:"Add State(s) to Queue__JKI_lib_State_Machine.vi"("State(s) in Front (\"\")"=w225, "State(s) in (\"\")"=w226) -> ("States Out"=w227:string)  [unwired: 13 in]
      }
      frame "API: Test SyncMessage With Error" {
        n99 = call "CSM - Check If Module Exists.vi"("CSM Name"=w241) -> ("error out"=w235:errorcluster, "Exist?"=w236:bool, "CSM Name (Dup)"=w240:string)  [unwired: 8 in]
        n100 = case shown="True" w236 {
          tunnel: w240 -> [_ w244]
          tunnel: [_ w243] -> w237
          frame False {
          }
          frame True {
            n101 = call "uuid.vi"() -> ("UUID"=w245:string)  [unwired: 11 in]
            n102 = call "Build Synchronous Message with Arguments.vi"("State With Arguments"="Message With Error", "Arguments (\"\")"=w245, "Target Module (\"\")"=w244) -> ("CSM Message String"=w243:string)  [unwired: 12 in]
          }
        }
        n103 = call <vilib>:"Add State(s) to Queue__JKI_lib_State_Machine.vi"("State(s) in Front (\"\")"=w237, "State(s) in (\"\")"=w238) -> ("States Out"=w239:string)  [unwired: 13 in]
      }
      frame "API: Test SyncMessage via API" {
        n104 = call "CSM - Check If Module Exists.vi"("CSM Name"=w269) -> ("error out"=w264:errorcluster, "Exist?"=w265:bool, "CSM Name (Dup)"=w268:string)  [unwired: 8 in]
        n105 = case shown="True" w265 {
          tunnel: w268 -> [_ w277]
          tunnel: [_ w276] -> w252
          tunnel: w254 -> [_ w275]
          tunnel: [_ w274] -> w261
          tunnel: [_ w273] -> w250
          tunnel: [_ w272] -> w257
          tunnel: [_ w271] -> w260
          frame False {
          }
          frame True {
            w274 = "Message" ("State With Arguments")
            n106 = call "uuid.vi"() -> ("UUID"=w272:string)  [unwired: 11 in]
            n107 = call "CSM - Wait and Send Message for Reply.vi"("State"=w274, "Current Module (\"\" to Generate an ID)"=w275, "Arguments (\"\")"=w272, "Target Module"=w277) -> ("Response"=w271:string, "Source CSM"=w273:string, "error out"=w276:errorcluster)  [unwired: 8 in, 1 out]
          }
        }
        n108 = call "Strip CSM name.vi"("CSM name"=w254) -> ("error out"=w251:errorcluster, "CSM name core"=w253:string)  [unwired: 7 in, 2 out]
        n109 = call "Strip CSM name.vi"("CSM name"=w250) -> ("error out"=w247:errorcluster, "CSM name core"=w249:string)  [unwired: 7 in, 2 out]
        n110 = Bundle By Name(cluster=T1 {"Arguments"="", "Response"="", "error"={"status"=FALSE, "code"=0, "source"=""}}, "Arguments"=w257, "Response"=w260, "error"=w252) -> (w255:T1)
        n111 = Concatenate Strings(w249, ":" ("string"), w261) -> (w259:string)
        n112 = Merge Errors(w251, w247) -> (w248:errorcluster)
        n113 = call "CSM - Set Module Attribute.vi"("CSM Name"=w253, "Attribute"=w259, "Value"=w255, "Error In"=w248) -> ("error out"=w258:errorcluster)  [unwired: 8 in, 3 out]
        n114 = call <vilib>:"Add State(s) to Queue__JKI_lib_State_Machine.vi"("State(s) in (\"\")"=w266) -> ("States Out"=w267:string)  [unwired: 14 in]
        n115 = Merge Errors(w258, w252, w264) -> (w263:errorcluster)
      }
      frame "API: Test SyncMessage With Error via API" {
        n116 = call "CSM - Check If Module Exists.vi"("CSM Name"=w300) -> ("error out"=w295:errorcluster, "Exist?"=w296:bool, "CSM Name (Dup)"=w299:string)  [unwired: 8 in]
        n117 = case shown="True" w296 {
          tunnel: w299 -> [_ w308]
          tunnel: [_ w307] -> w282
          tunnel: w285 -> [_ w306]
          tunnel: [_ w305] -> w292
          tunnel: [_ w304] -> w281
          tunnel: [_ w303] -> w288
          tunnel: [_ w302] -> w291
          frame False {
          }
          frame True {
            w305 = "Message With Error" ("State With Arguments")
            n118 = call "uuid.vi"() -> ("UUID"=w303:string)  [unwired: 11 in]
            n119 = call "CSM - Wait and Send Message for Reply.vi"("State"=w305, "Current Module (\"\" to Generate an ID)"=w306, "Arguments (\"\")"=w303, "Target Module"=w308) -> ("Response"=w302:string, "Source CSM"=w304:string, "error out"=w307:errorcluster)  [unwired: 8 in, 1 out]
          }
        }
        n120 = call "Strip CSM name.vi"("CSM name"=w281) -> ("error out"=w278:errorcluster, "CSM name core"=w280:string)  [unwired: 7 in, 2 out]
        n121 = Bundle By Name(cluster=T1 {"Arguments"="", "Response"="", "error"={"status"=FALSE, "code"=0, "source"=""}}, "Arguments"=w288, "Response"=w291, "error"=w282) -> (w287:T1)
        n122 = call "Strip CSM name.vi"("CSM name"=w285) -> ("error out"=w283:errorcluster, "CSM name core"=w284:string)  [unwired: 7 in, 2 out]
        n123 = Concatenate Strings(w280, ":" ("string"), w292) -> (w290:string)
        n124 = Merge Errors(w283, w278) -> (w279:errorcluster)
        n125 = call "CSM - Set Module Attribute.vi"("CSM Name"=w284, "Attribute"=w290, "Value"=w287, "Error In"=w279) -> ("error out"=w289:errorcluster)  [unwired: 8 in, 3 out]
        n126 = call <vilib>:"Add State(s) to Queue__JKI_lib_State_Machine.vi"("State(s) in (\"\")"=w297) -> ("States Out"=w298:string)  [unwired: 14 in]
        n127 = Merge Errors(w289, w282, w295) -> (w294:errorcluster)
      }
      frame "API: Test AsyncMessageWithReply" {
        n128 = call "CSM - Check If Module Exists.vi"("CSM Name"=w315) -> ("error out"=w309:errorcluster, "Exist?"=w310:bool, "CSM Name (Dup)"=w314:string)  [unwired: 8 in]
        n129 = case shown="True" w310 {
          tunnel: w314 -> [_ w318]
          tunnel: [_ w317] -> w311
          frame False {
          }
          frame True {
            n130 = call "uuid.vi"() -> ("UUID"=w319:string)  [unwired: 11 in]
            n131 = call-poly "Build Message with Arguments++.vi"("State With Arguments"="Message", "Arguments (\"\")"=w319, "Target Module (\"\")"=w318) -> ("CSM Message String"=w317:string)  [unwired: 12 in]
          }
        }
        n132 = call <vilib>:"Add State(s) to Queue__JKI_lib_State_Machine.vi"("State(s) in Front (\"\")"=w311, "State(s) in (\"\")"=w312) -> ("States Out"=w313:string)  [unwired: 13 in]
      }
      frame "API: Test AsyncMessageWithReply With Error" {
        n133 = call "CSM - Check If Module Exists.vi"("CSM Name"=w327) -> ("error out"=w321:errorcluster, "Exist?"=w322:bool, "CSM Name (Dup)"=w326:string)  [unwired: 8 in]
        n134 = case shown="True" w322 {
          tunnel: w326 -> [_ w331]
          tunnel: [_ w329] -> w323
          frame False {
          }
          frame True {
            n135 = call "uuid.vi"() -> ("UUID"=w330:string)  [unwired: 11 in]
            n136 = call-poly "Build Message with Arguments++.vi"("State With Arguments"="Message With Error", "Arguments (\"\")"=w330, "Target Module (\"\")"=w331) -> ("CSM Message String"=w329:string)  [unwired: 12 in]
          }
        }
        n137 = call <vilib>:"Add State(s) to Queue__JKI_lib_State_Machine.vi"("State(s) in Front (\"\")"=w323, "State(s) in (\"\")"=w324) -> ("States Out"=w325:string)  [unwired: 13 in]
      }
      frame "API: Test AsyncMessageWithoutReply" {
        n138 = call "CSM - Check If Module Exists.vi"("CSM Name"=w339) -> ("error out"=w333:errorcluster, "Exist?"=w334:bool, "CSM Name (Dup)"=w338:string)  [unwired: 8 in]
        n139 = case shown="True" w334 {
          tunnel: w338 -> [_ w344]
          tunnel: [_ w342] -> w335
          frame False {
          }
          frame True {
            n140 = call-poly "Build Message with Arguments++.vi"("State With Arguments"="AsyncMessageWithoutReply", "Arguments (\"\")"="123456789" ("Arguments (\"\")"), "Target Module (\"\")"=w344) -> ("CSM Message String"=w342:string)  [unwired: 12 in]
          }
        }
        n141 = call <vilib>:"Add State(s) to Queue__JKI_lib_State_Machine.vi"("State(s) in Front (\"\")"=w335, "State(s) in (\"\")"=w336) -> ("States Out"=w337:string)  [unwired: 13 in]
      }
      frame "API: Test AsyncMessageWithoutReply via API" {
        n142 = call "CSM - Check If Module Exists.vi"("CSM Name"=w353) -> ("error out"=w348:errorcluster, "Exist?"=w349:bool, "CSM Name (Dup)"=w352:string)  [unwired: 8 in]
        n143 = case shown="True" w349 {
          tunnel: w352 -> [_ w356]
          tunnel: w347 -> [_ w359]
          tunnel: [_ w355] -> w345
          frame False {
          }
          frame True {
            n144 = call "CSM - Wait and Post Message.vi"("State"="AsyncMessageWithoutReply" ("State With Arguments"), "Current Module (\"\" to Generate an ID)"=w359, "Arguments (\"\")"="123456789" ("Arguments (\"\")"), "Target Module"=w356) -> ("error out"=w355:errorcluster)  [unwired: 10 in, 1 out]
          }
        }
        n145 = call <vilib>:"Add State(s) to Queue__JKI_lib_State_Machine.vi"("State(s) in (\"\")"=w350) -> ("States Out"=w351:string)  [unwired: 14 in]
        n146 = Merge Errors(w345, w348) -> (w346:errorcluster)
      }
      frame "API: Test Argument" {
        n147 = call "uuid.vi"() -> ("UUID"=w365:string)  [unwired: 11 in]
        n148 = call "CSM - Convert HexStr to Data.vi"("HEX String"=w369) -> ("Variant"=w367:variant, "error out"=w368:errorcluster)  [unwired: 7 in]
        n149 = Bundle("", "UUID"=w365) -> (w363:cluster{string, "UUID":string})  [unwired: 1 in]
        n150 = Variant To Data(error in=w368, type=w363, Variant=w367) -> (data=w362:cluster{string, "UUID":string}, error out=w366:errorcluster)
        n151 = Unbundle(w362) -> (w361:string, "UUID"=w360:string)
        n152 = call "CSM - Check If Module Exists.vi"("Error In"=w366, "CSM Name"=w361) -> ("error out"=w370:errorcluster, "Exist?"=w371:bool, "CSM Name (Dup)"=w375:string)  [unwired: 7 in]
        n153 = case shown="True" w371 {
          tunnel: w375 -> [_ w379]
          tunnel: [_ w378] -> w372
          tunnel: w360 -> [_ w377]
          frame False {
          }
          frame True {
            n154 = call "Build Synchronous Message with Arguments.vi"("State With Arguments"="ArgumentTest", "Arguments (\"\")"=w377, "Target Module (\"\")"=w379) -> ("CSM Message String"=w378:string)  [unwired: 12 in]
          }
        }
        n155 = call <vilib>:"Add State(s) to Queue__JKI_lib_State_Machine.vi"("State(s) in Front (\"\")"=w372, "State(s) in (\"\")"=w373) -> ("States Out"=w374:string)  [unwired: 13 in]
      }
      frame "API: Test Argument Only For Chain4", "API: Test Argument Only For Chain4And5", "API: Test Argument Only For Chain4And5And6", "API: Test Argument Only For Chain4And6", "API: Test Argument Only For Chain5", "API: Test Argument Only For Chain5And6", "API: Test Argument Only For Chain6" {
        n156 = call "uuid.vi"() -> ("UUID"=w399:string)  [unwired: 11 in]
        n157 = call "CSM - Convert HexStr to Data.vi"("HEX String"=w403) -> ("Variant"=w401:variant, "error out"=w402:errorcluster)  [unwired: 7 in]
        n158 = Match Pattern(string=w387, regular expression="Chain") -> (after substring=w382:string, offset past match=w385:i32)  [unwired: 1 in, 2 out]
        n159 = Bundle("", "UUID"=w399) -> (w397:cluster{string, "UUID":string})  [unwired: 1 in]
        n160 = Variant To Data(error in=w402, type=w397, Variant=w401) -> (data=w396:cluster{string, "UUID":string}, error out=w400:errorcluster)
        n161 = Not Equal?(x=w385, y=-1) -> (x != y?=w383:bool)
        n162 = call "CSM - Resolve Node Module.vi"("Node Name"=w393) -> ("CSM Module Name"=w392:string)  [unwired: 10 in]
        n163 = case shown="True" w383 {
          tunnel: w382 -> [_ w409]
          tunnel: [_ w409] -> w381
          frame False {
          }
          frame True {
          }
        }
        n164 = Unbundle(w396) -> (w395:string, "UUID"=w394:string)
        n165 = call "CSM - Check If Module Exists.vi"("Error In"=w400, "CSM Name"=w395) -> ("error out"=w391:errorcluster, "Exist?"=w404:bool, "CSM Name (Dup)"=w407:string)  [unwired: 7 in]
        n166 = case shown="True" w404 {
          tunnel: w407 -> [_ w416]
          tunnel: w394 -> [_ w417]
          tunnel: [_ w415] -> w388
          tunnel: w392 -> [_ w414]
          tunnel: [_ w413] -> w390
          tunnel: w381 -> [_ w411]
          frame False {
          }
          frame True {
            n167 = Concatenate Strings("ArgumentTestOnlyForChain" ("State With Arguments"), w411) -> (w410:string)
            n168 = call "CSM - Wait and Send Message for Reply.vi"("State"=w410, "Current Module (\"\" to Generate an ID)"=w414, "Arguments (\"\")"=w417, "Target Module"=w416) -> ("Response"=w413:string, "error out"=w415:errorcluster)  [unwired: 8 in, 2 out]
          }
        }
        n169 = call <vilib>:"Add State(s) to Queue__JKI_lib_State_Machine.vi"("State(s) in (\"\")"=w405) -> ("States Out"=w406:string)  [unwired: 14 in]
        n170 = Merge Errors(w391, w388) -> (w389:errorcluster)
      }
      frame "API: Test Response With Error" {
        n171 = call "CSM - Check If Module Exists.vi"("CSM Name"=w424) -> ("error out"=w418:errorcluster, "Exist?"=w419:bool, "CSM Name (Dup)"=w423:string)  [unwired: 8 in]
        n172 = case shown="True" w419 {
          tunnel: w423 -> [_ w427]
          tunnel: [_ w426] -> w420
          frame False {
          }
          frame True {
            n173 = call "uuid.vi"() -> ("UUID"=w428:string)  [unwired: 11 in]
            n174 = call "Build Synchronous Message with Arguments.vi"("State With Arguments"="Response With Error", "Arguments (\"\")"=w428, "Target Module (\"\")"=w427) -> ("CSM Message String"=w426:string)  [unwired: 12 in]
          }
        }
        n175 = call <vilib>:"Add State(s) to Queue__JKI_lib_State_Machine.vi"("State(s) in Front (\"\")"=w420, "State(s) in (\"\")"=w421) -> ("States Out"=w422:string)  [unwired: 13 in]
      }
      frame "API: Test MacroWithSubMessages" {
        n176 = call <vilib>:"Build State String with Arguments__JKI_lib_State_Machine.vi"("Arguments (\"\")"=w431, "State"="Macro: Test MacroWithSubMessages") -> ("State with Arguments"=w430:string)  [unwired: 4 in]
        n177 = call <vilib>:"Add State(s) to Queue__JKI_lib_State_Machine.vi"("State(s) in Front (\"\")"=w430, "State(s) in (\"\")"=w434) -> ("States Out"=w433:string)  [unwired: 13 in]
      }
      frame "API: Test MacroWithSubAndPostMessages" {
        n178 = call <vilib>:"Build State String with Arguments__JKI_lib_State_Machine.vi"("Arguments (\"\")"=w438, "State"="Macro: Test MacroWithSubAndPostMessages") -> ("State with Arguments"=w437:string)  [unwired: 4 in]
        n179 = call <vilib>:"Add State(s) to Queue__JKI_lib_State_Machine.vi"("State(s) in Front (\"\")"=w437, "State(s) in (\"\")"=w441) -> ("States Out"=w440:string)  [unwired: 13 in]
      }
      frame "API: Test MacroWithNonLocalSubMessages" {
        n180 = call <vilib>:"Build State String with Arguments__JKI_lib_State_Machine.vi"("Arguments (\"\")"=w445, "State"="Macro: TestMacroWithNonLocalSubMessages") -> ("State with Arguments"=w444:string)  [unwired: 4 in]
        n181 = call <vilib>:"Add State(s) to Queue__JKI_lib_State_Machine.vi"("State(s) in Front (\"\")"=w444, "State(s) in (\"\")"=w448) -> ("States Out"=w447:string)  [unwired: 13 in]
      }
      frame "API: Test Register State" {
        n182 = call <vilib>:"Build State String with Arguments__JKI_lib_State_Machine.vi"("Arguments (\"\")"=w452, "State"="Test Status") -> ("State with Arguments"=w451:string)  [unwired: 4 in]
        n183 = call <vilib>:"Add State(s) to Queue__JKI_lib_State_Machine.vi"("State(s) in Front (\"\")"=w451, "State(s) in (\"\")"=w455) -> ("States Out"=w454:string)  [unwired: 13 in]
      }
      frame "API: Test Register State Argument Info" {
        n184 = call <vilib>:"Build State String with Arguments__JKI_lib_State_Machine.vi"("Arguments (\"\")"=w459, "State"="Register State Argument Info") -> ("State with Arguments"=w458:string)  [unwired: 4 in]
        n185 = call <vilib>:"Add State(s) to Queue__JKI_lib_State_Machine.vi"("State(s) in Front (\"\")"=w458, "State(s) in (\"\")"=w462) -> ("States Out"=w461:string)  [unwired: 13 in]
      }
      frame "API: Test Register Status" {
        n186 = call <vilib>:"Build State String with Arguments__JKI_lib_State_Machine.vi"("Arguments (\"\")"=w466, "State"="Register Status") -> ("State with Arguments"=w465:string)  [unwired: 4 in]
        n187 = call <vilib>:"Add State(s) to Queue__JKI_lib_State_Machine.vi"("State(s) in Front (\"\")"=w465, "State(s) in (\"\")"=w469) -> ("States Out"=w468:string)  [unwired: 13 in]
      }
      frame "API: Test Register Interrupt" {
        n188 = call <vilib>:"Build State String with Arguments__JKI_lib_State_Machine.vi"("Arguments (\"\")"=w473, "State"="Register Interrupt") -> ("State with Arguments"=w472:string)  [unwired: 4 in]
        n189 = call <vilib>:"Add State(s) to Queue__JKI_lib_State_Machine.vi"("State(s) in Front (\"\")"=w472, "State(s) in (\"\")"=w476) -> ("States Out"=w475:string)  [unwired: 13 in]
      }
      frame "API: Test Register Status Argument Info" {
        n190 = call <vilib>:"Build State String with Arguments__JKI_lib_State_Machine.vi"("Arguments (\"\")"=w480, "State"="Register Status Argument Info") -> ("State with Arguments"=w479:string)  [unwired: 4 in]
        n191 = call <vilib>:"Add State(s) to Queue__JKI_lib_State_Machine.vi"("State(s) in Front (\"\")"=w479, "State(s) in (\"\")"=w483) -> ("States Out"=w482:string)  [unwired: 13 in]
      }
      frame "API: Test Status A" {
        n192 = call <vilib>:"Build State String with Arguments__JKI_lib_State_Machine.vi"("Arguments (\"\")"=w487, "State"="Broadcast Status A") -> ("State with Arguments"=w488:string)  [unwired: 4 in]
        n193 = call <vilib>:"Add State(s) to Queue__JKI_lib_State_Machine.vi"("State(s) in Front (\"\")"=w488, "State(s) in (\"\")"=w490) -> ("States Out"=w489:string)  [unwired: 13 in]
      }
      frame "API: Test State A" {
        n194 = call <vilib>:"Build State String with Arguments__JKI_lib_State_Machine.vi"("Arguments (\"\")"=w494, "State"="State A") -> ("State with Arguments"=w495:string)  [unwired: 4 in]
        n195 = call <vilib>:"Add State(s) to Queue__JKI_lib_State_Machine.vi"("State(s) in Front (\"\")"=w495, "State(s) in (\"\")"=w497) -> ("States Out"=w496:string)  [unwired: 13 in]
      }
      frame "API: Test State B" {
        n196 = call <vilib>:"Build State String with Arguments__JKI_lib_State_Machine.vi"("Arguments (\"\")"=w501, "State"="State B") -> ("State with Arguments"=w502:string)  [unwired: 4 in]
        n197 = call <vilib>:"Add State(s) to Queue__JKI_lib_State_Machine.vi"("State(s) in Front (\"\")"=w502, "State(s) in (\"\")"=w504) -> ("States Out"=w503:string)  [unwired: 13 in]
      }
      frame "API: Test Status B" {
        n198 = call <vilib>:"Build State String with Arguments__JKI_lib_State_Machine.vi"("Arguments (\"\")"=w508, "State"="Broadcast Status B") -> ("State with Arguments"=w509:string)  [unwired: 4 in]
        n199 = call <vilib>:"Add State(s) to Queue__JKI_lib_State_Machine.vi"("State(s) in Front (\"\")"=w509, "State(s) in (\"\")"=w511) -> ("States Out"=w510:string)  [unwired: 13 in]
      }
      frame "API: Local Registration" {
        # "Test Status @ From >> Handler Message @ To -><register>"
        n200 = call "Strip CSM name.vi"("CSM name"=w519) -> ("error out"=w517:errorcluster, "CSM name core"=w514:string)  [unwired: 7 in, 2 out]
        n201 = call-poly "Build Message with Arguments++.vi"("Target CSM"=w515, "Source CSM (* as Default)"=w514, "Status"="Test Status", "API (If \"\", Same As \"Status\")"="Handler Message") -> ("CSM Message String"=w516:string)  [unwired: 11 in]
        n202 = call <vilib>:"Add State(s) to Queue__JKI_lib_State_Machine.vi"("State(s) in Front (\"\")"=w516, "State(s) in (\"\")"=w523) -> ("States Out"=w522:string)  [unwired: 13 in]
      }
      frame "API: Local Registration II" {
        # "Test Status @ From >> Handler Message -><register>"
        n203 = call "Strip CSM name.vi"("CSM name"=w528) -> ("error out"=w526:errorcluster, "CSM name core"=w524:string)  [unwired: 7 in, 2 out]
        n204 = call-poly "Build Message with Arguments++.vi"("Source CSM (* as Default)"=w524, "Status"="Test Status", "API (If \"\", Same As \"Status\")"="Handler Message") -> ("CSM Message String"=w525:string)  [unwired: 12 in]
        n205 = call <vilib>:"Add State(s) to Queue__JKI_lib_State_Machine.vi"("State(s) in Front (\"\")"=w525, "State(s) in (\"\")"=w532) -> ("States Out"=w531:string)  [unwired: 13 in]
      }
      frame "API: Local Unregistration" {
        # "Test Status @ From >> Handler Message @ To -><unregister>"
        n206 = call "Strip CSM name.vi"("CSM name"=w538) -> ("error out"=w536:errorcluster, "CSM name core"=w533:string)  [unwired: 7 in, 2 out]
        n207 = call-poly "Build Message with Arguments++.vi"("Target CSM"=w534, "Source CSM (* as Default)"=w533, "Status"="Test Status", "API (If \"\", Same As \"Status\")"="Handler Message") -> ("CSM Message String"=w535:string)  [unwired: 11 in]
        n208 = call <vilib>:"Add State(s) to Queue__JKI_lib_State_Machine.vi"("State(s) in Front (\"\")"=w535, "State(s) in (\"\")"=w542) -> ("States Out"=w541:string)  [unwired: 13 in]
      }
      frame "API: Local Registration via API" {
        # "Test Status @ From >> Handler Message @ To -><register>"
        n209 = call "Strip CSM name.vi"("CSM name"=w549) -> ("error out"=w548:errorcluster, "CSM name core"=w544:string)  [unwired: 7 in, 2 out]
        n210 = call "CSM - Register Broadcast.vi"("CSM Name(Empty for Broadcast Event)"=w543, "Source CSM Name (* as Default)"=w544, "Trigger"="Test Status", "API (If \"\", Same as Trigger)"="Handler Message", "Error In"=w548) -> ("error out"=w547:errorcluster)  [unwired: 9 in, 1 out]
        n211 = call <vilib>:"Add State(s) to Queue__JKI_lib_State_Machine.vi"("State(s) in (\"\")"=w552) -> ("States Out"=w551:string)  [unwired: 14 in]
      }
      frame "API: Local Unregistration via API" {
        # "Test Status @ From >> Handler Message @ To -><unregister>"
        n212 = call "Strip CSM name.vi"("CSM name"=w559) -> ("error out"=w558:errorcluster, "CSM name core"=w554:string)  [unwired: 7 in, 2 out]
        n213 = call "CSM - Unregister Broadcast.vi"("CSM Name(Empty for Broadcast Event)"=w553, "Source CSM Name (* as Default)"=w554, "Trigger"="Test Status", "API (\"*\" as Default)"="Handler Message", "Error In"=w558) -> ("error out"=w557:errorcluster)  [unwired: 9 in, 1 out]
        n214 = call <vilib>:"Add State(s) to Queue__JKI_lib_State_Machine.vi"("State(s) in (\"\")"=w562) -> ("States Out"=w561:string)  [unwired: 14 in]
      }
      frame "API: API2" {
        # "#CSM API Example\nCopy/Rename this case for your own API"
        # "unpack Hex String  to Variant\nif complex parameter is needed."
        n215 = call "CSM - Convert HexStr to Data.vi"("HEX String"=w564) -> ()  [unwired: 7 in, 2 out]
        n216 = disable-structure shown="Enabled" {
          disable-tunnel: [w567 "API2 Response"] -> w563
          frame Disabled {
            # "pack variant to hexstr \nif complex response is needed."
            # "complex Response"
            n217 = call "CSM - Convert Data to HexStr.vi"() -> ("HEX String (0-9,A-F)"=w567:string)  [unwired: 9 in]
          }
          frame Enabled {
          }
        }
      }
      frame "---------- Action ----------" {
        # "#CSM \"Category Seperator\"\nDo not put any code in this frame."
        n218 = call <vilib>:"Add State(s) to Queue__JKI_lib_State_Machine.vi"("State(s) in (\"\")"=w571) -> ("States Out"=w570:string)  [unwired: 14 in]
      }
      frame "Action: action1" {
        # "#CSM \"Internal State\"\nThis category is used for holding internal states"
        n219 = call <vilib>:"Add State(s) to Queue__JKI_lib_State_Machine.vi"("State(s) in (\"\")"=w574) -> ("States Out"=w573:string)  [unwired: 14 in]
      }
      frame "Test Status" {
        n220 = call <vilib>:"Add State(s) to Queue__JKI_lib_State_Machine.vi"("State(s) in (\"\")"=w578) -> ("States Out"=w577:string)  [unwired: 14 in]
      }
      frame "Register State Argument Info" {
        n221 = call "Strip CSM name.vi"("CSM name"=w582) -> ("error out"=w581:errorcluster, "CSM name core"=w583:string)  [unwired: 7 in, 2 out]
        n222 = Concatenate Strings(w579, "+", w583) -> (w580:string)
        n223 = call <vilib>:"Add State(s) to Queue__JKI_lib_State_Machine.vi"("State(s) in (\"\")"=w585) -> ("States Out"=w587:string)  [unwired: 14 in]
      }
      frame "Register Status" {
        n224 = call <vilib>:"Build State String with Arguments__JKI_lib_State_Machine.vi"("Arguments (\"\")"=w588, "State"="Test Status") -> ("State with Arguments"=w590:string)  [unwired: 4 in]
        n225 = call "CSM - Broadcast Status Change.vi"("Status With Arguments"=w590, "State Queue"=w592) -> ("Remaining States"=w589:string)  [unwired: 13 in]
      }
      frame "Register Interrupt" {
        n226 = call-poly "Build Message with Arguments++.vi"("State With Arguments"="Test Interrupt", "Arguments (\"\")"=w597) -> ("CSM Message String"=w596:string)  [unwired: 13 in]
        n227 = call <vilib>:"Add State(s) to Queue__JKI_lib_State_Machine.vi"("State(s) in Front (\"\")"=w596, "State(s) in (\"\")"=w595) -> ("States Out"=w594:string)  [unwired: 13 in]
      }
      frame "Register Status Argument Info" {
        w605 = "Test Status Argument Info"
        n228 = call "Strip CSM name.vi"("CSM name"=w603) -> ("error out"=w601:errorcluster, "CSM name core"=w602:string)  [unwired: 7 in, 2 out]
        n229 = Concatenate Strings(w605, "+", w602) -> (w600:string)
        n230 = call <vilib>:"Build State String with Arguments__JKI_lib_State_Machine.vi"("Arguments (\"\")"=w600, "State"=w605) -> ("State with Arguments"=w607:string)  [unwired: 4 in]
        n231 = call "CSM - Broadcast Status Change.vi"("Status With Arguments"=w607, "State Queue"=w608) -> ("Remaining States"=w606:string)  [unwired: 13 in]
      }
      frame "Broadcast Status A" {
        n232 = call <vilib>:"Build State String with Arguments__JKI_lib_State_Machine.vi"("Arguments (\"\")"=w610, "State"="Status A") -> ("State with Arguments"=w612:string)  [unwired: 4 in]
        n233 = call "CSM - Broadcast Status Change.vi"("Status With Arguments"=w612, "State Queue"=w614) -> ("Remaining States"=w611:string)  [unwired: 13 in]
      }
      frame "Broadcast Status B" {
        n234 = call <vilib>:"Build State String with Arguments__JKI_lib_State_Machine.vi"("Arguments (\"\")"=w616, "State"="Status B") -> ("State with Arguments"=w618:string)  [unwired: 4 in]
        n235 = call "CSM - Broadcast Status Change.vi"("Status With Arguments"=w618, "State Queue"=w620) -> ("Remaining States"=w617:string)  [unwired: 13 in]
      }
      frame "State A" {
        n236 = call <vilib>:"Add State(s) to Queue__JKI_lib_State_Machine.vi"("State(s) in (\"\")"=w624) -> ("States Out"=w623:string)  [unwired: 14 in]
      }
      frame "State B" {
        n237 = call <vilib>:"Add State(s) to Queue__JKI_lib_State_Machine.vi"("State(s) in (\"\")"=w629) -> ("States Out"=w628:string)  [unwired: 14 in]
      }
      frame "Message" {
      }
      frame "SubMessage1" {
      }
      frame "SubMessage2" {
      }
      frame "SubMessage3" {
        n238 = call "Strip CSM name.vi"("CSM name"=w650) -> ("error out"=w648:errorcluster, "CSM name core"=w649:string)  [unwired: 7 in, 2 out]
        n239 = call "CSM - Set Module Attribute.vi"("CSM Name"=w649, "Attribute"=w647, "Value"=w646, "Error In"=w648) -> ("error out"=w644:errorcluster)  [unwired: 8 in, 3 out]
        n240 = Merge Errors(w644, w653) -> (w645:errorcluster)
      }
      frame "PostMessage1" {
      }
      frame "Message With Error" {
        n241 = Merge Errors(errorcluster {"status"=TRUE, "code"=1234567898, "source"="Simulated Error\nwill be sent to Response case"} ("error out"), w659) -> (w658:errorcluster)
      }
      frame "Response With Error" {
        n242 = Merge Errors(errorcluster {"status"=TRUE, "code"=1234567898, "source"="Simulated Error"} ("error out"), w665) -> (w664:errorcluster)
      }
      frame "ArgumentTest" {
        n243 = call "Strip CSM name.vi"("CSM name"=w676) -> ("error out"=w673:errorcluster, "CSM name core"=w675:string)  [unwired: 7 in, 2 out]
        n244 = call "CSM - Set Module Attribute.vi"("CSM Name"=w675, "Attribute"=w672, "Value"=w674, "Error In"=w673) -> ("error out"=w670:errorcluster)  [unwired: 8 in, 3 out]
        n245 = Merge Errors(w670, w679) -> (w671:errorcluster)
      }
      frame "ArgumentTestOnlyForChain4", "ArgumentTestOnlyForChain4And5", "ArgumentTestOnlyForChain4And5And6", "ArgumentTestOnlyForChain4And6", "ArgumentTestOnlyForChain5", "ArgumentTestOnlyForChain5And6", "ArgumentTestOnlyForChain6" {
        n246 = call "Strip CSM name.vi"("CSM name"=w680) -> ("error out"=w685:errorcluster, "CSM name core"=w686:string)  [unwired: 7 in, 2 out]
        n247 = call "CSM - Set Module Attribute.vi"("CSM Name"=w686, "Attribute"=w680, "Value"=w680, "Error In"=w685) -> ("error out"=w682:errorcluster)  [unwired: 8 in, 3 out]
        n248 = Merge Errors(w682, w688) -> (w684:errorcluster)
      }
      frame "AsyncMessageWithoutReply" {
        # "123456789 string constant"
        n249 = call "Strip CSM name.vi"("CSM name"=w693) -> ("error out"=w691:errorcluster, "CSM name core"=w692:string)  [unwired: 7 in, 2 out]
        n250 = call "CSM - Set Module Attribute.vi"("CSM Name"=w692, "Attribute"=w694, "Value"=w695, "Error In"=w691) -> ("error out"=w689:errorcluster)  [unwired: 8 in, 3 out]
        n251 = Merge Errors(w689, w698) -> (w690:errorcluster)
      }
      frame "Handler Message" {
        n252 = call "Strip CSM name.vi"("CSM name"=w705) -> ("error out"=w703:errorcluster, "CSM name core"=w704:string)  [unwired: 7 in, 2 out]
        n253 = call "CSM - Set Module Attribute.vi"("CSM Name"=w704, "Attribute"=w701, "Value"=w700, "Error In"=w703) -> ("error out"=w699:errorcluster)  [unwired: 8 in, 3 out]
        n254 = Merge Errors(w708, w699) -> (w702:errorcluster)
      }
      frame "Handler Message With Counter" {
        n255 = Unbundle By Name(w714) -> ("Counter"=w715:u32)
        n256 = Decimal String To Number(string=w712) -> (number=w709:i32)  [unwired: 2 in, 1 out]
        n257 = Increment(x=w715) -> (x+1=w710:u32)
        n258 = Bundle By Name(cluster=w714, "Counter"=w710) -> (w713:T6)
        n259 = Equal?(x=w710, y=w709) -> (x = y?=w711:bool)
        n260 = call "Strip CSM name.vi"("CSM name"=w721) -> ("error out"=w719:errorcluster, "CSM name core"=w720:string)  [unwired: 7 in, 2 out]
        n261 = case shown="True" w711 {
          tunnel: w720 -> [_ w729]
          tunnel: w719 -> [w724 w728]
          tunnel: w717 -> [_ w727]
          tunnel: [w724 w726] -> w716
          tunnel: w710 -> [_ w725]
          frame False {
          }
          frame True {
            n262 = call "CSM - Set Module Attribute.vi"("CSM Name"=w729, "Attribute"=w727, "Value"=w725, "Error In"=w728) -> ("error out"=w726:errorcluster)  [unwired: 8 in, 3 out]
          }
        }
        n263 = Merge Errors(w723, w716) -> (w718:errorcluster)
      }
      frame "Reset Counter" {
        # "#CSM \"Internal State\"\nThis category is used for holding internal states"
        n264 = Bundle By Name(cluster=w732, "Counter"=u32 0) -> (w730:T6)
        n265 = call <vilib>:"Add State(s) to Queue__JKI_lib_State_Machine.vi"("State(s) in (\"\")"=w734) -> ("States Out"=w733:string)  [unwired: 14 in]
      }
    }
  }
